vi "ActiveObjects_DynamicEvents_ProcessRepository_EndevoGoop3.vi"(0 "reference in":refnum<class>, 1 "Action(ReadRepository)":T1(ring), 5 "error in (no error)":errorcluster) -> (7 "QueueFromProcess":refnum<queue>, 9 "ProcessViRef":refnum<vi>, 11 "ProcessSyncQueue":refnum<queue>, 13 "EventFromProcess":refnum<user-event>, 14 "reference out":refnum<class>, 15 "EventsToProcess":refnum<user-event>, 17 "ProcessAlreadyStarted":bool, 19 "error out":errorcluster)   [LabVIEW 2010]
uses:
  ActiveObjects_DynamicEvents_Process.ctl
panel:
  # "Use this indicator for sending messages to the Process VI"
  # "These indicators are used by the process VIs"
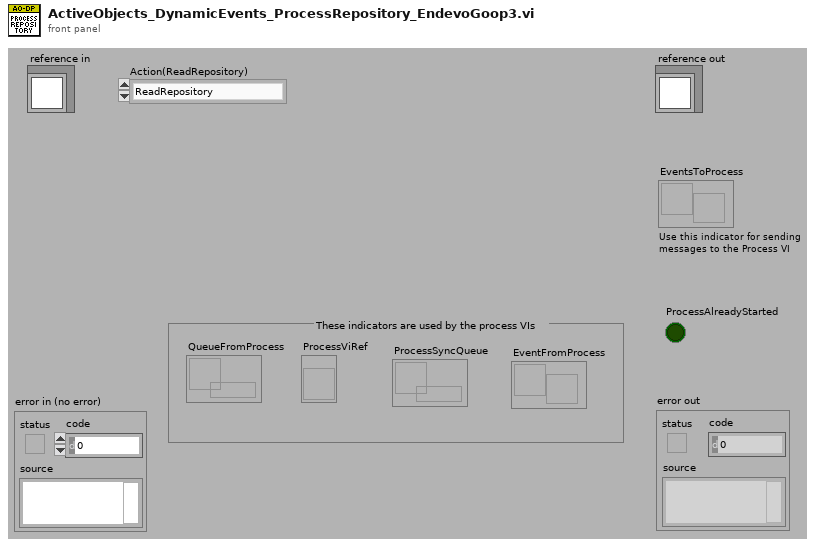
[diagram p1: front panel]
types:
  T1 = enum16{"ReadRepository", "CreateNew", "CreateOrLookUpExisting"}
  T2 = typedef "ActiveObjects_DynamicEvents_Process.ctl" = cluster{"EventsToProcess":refnum<user-event>, "EventFromProcess":refnum<user-event>, "ProcessSyncQueue":refnum<queue>, "ProcessViRef":refnum<vi>, "QueueFromProcess":refnum<queue>}
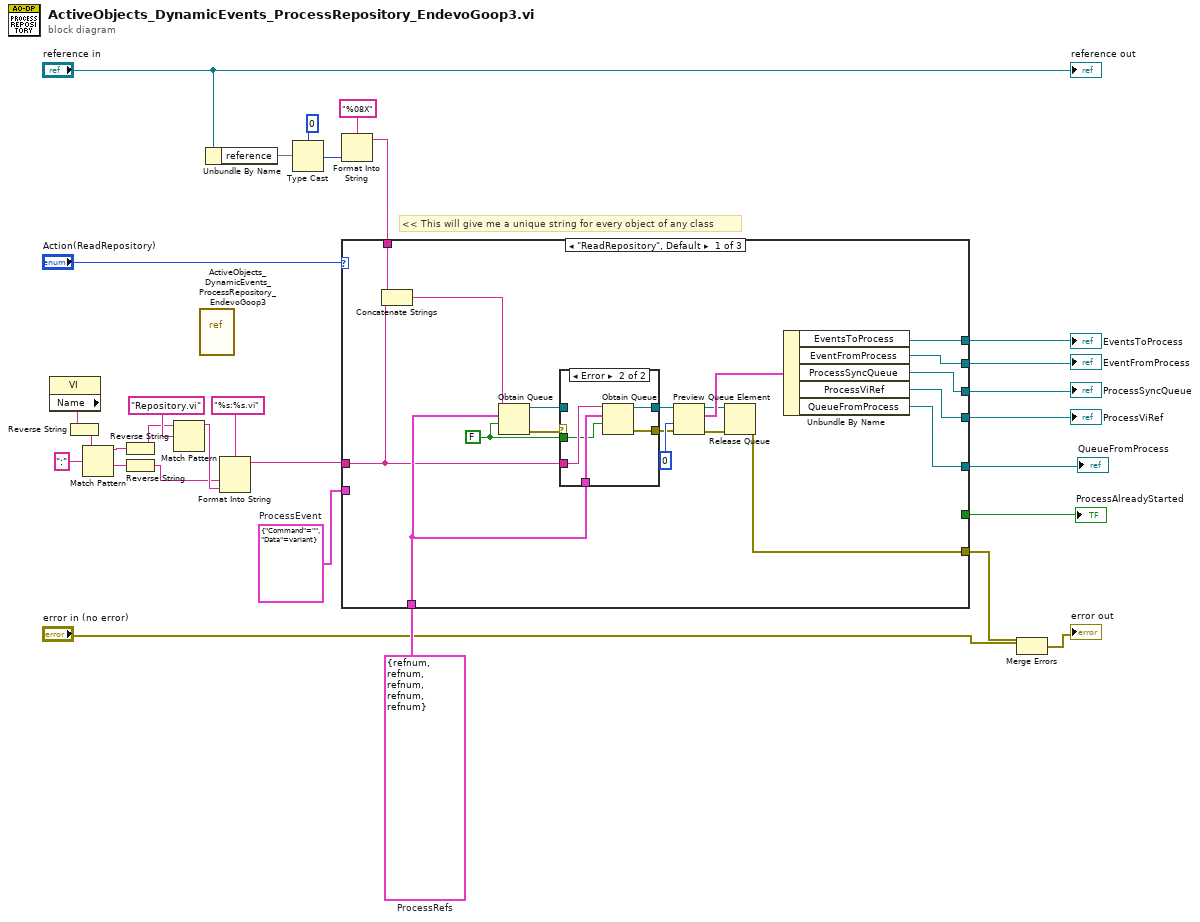
[diagram p0: block diagram]
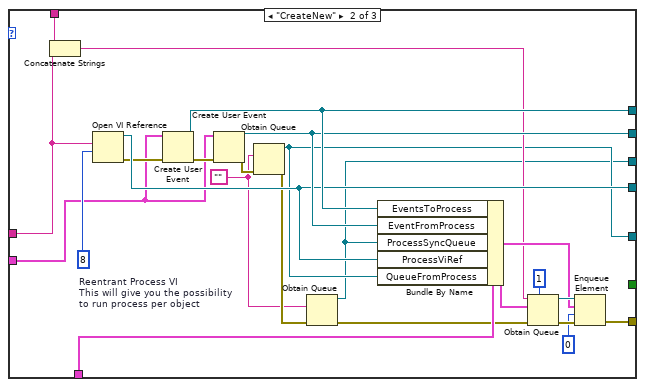
[diagram p3: hidden frame]
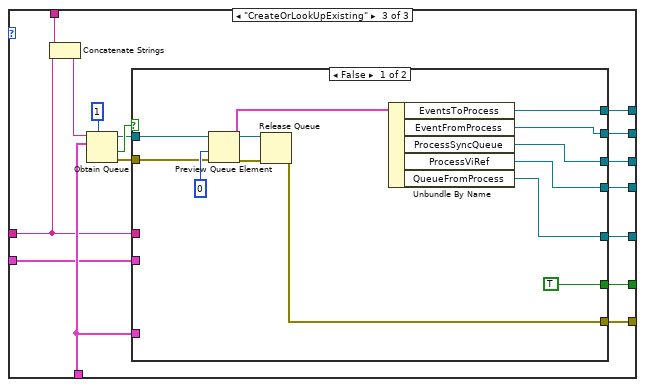
[diagram p4: hidden frame]
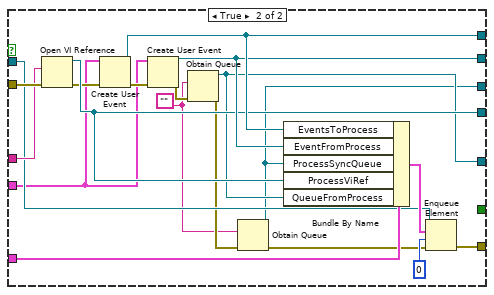
[diagram p5: hidden frame]
diagram:
  w13 = T2 {"EventsToProcess"=refnum, "EventFromProcess"=refnum, "ProcessSyncQueue"=refnum, "ProcessViRef"=refnum, "QueueFromProcess"=refnum}  # ProcessRefs
  w14 = cluster{"Command":string, "Data":variant} {"Command"="", "Data"=variant}  # ProcessEvent
  # "<< This will give me a unique string for every object of any class"
  n1 = property class="VI"() -> ("Name"=w20:string)  [unwired: 2 in, 2 out]
  n2 = Reverse String(1:w20) -> (0:w21:string)
  n3 = Match Pattern(string=w21, regular expression=":") -> (before substring=w25:string, after substring=w22:string)  [unwired: 1 in, 2 out]
  n4 = Reverse String(1:w25) -> (0:w26:string)
  n5 = Reverse String(1:w22) -> (0:w24:string)
  n6 = Match Pattern(string=w26, regular expression="Repository.vi") -> (before substring=w28:string)  [unwired: 1 in, 3 out]
  n7 = vi-ref "ActiveObjects_DynamicEvents_ProcessRepository_EndevoGoop3.vi"() -> ()  [unwired: 1 out]
  n8 = Unbundle By Name("reference in") -> ("reference"=w15)
  n9 = Format Into String(format string="%s:%s.vi", w24, w28) -> (resulting string=w3:string)  [unwired: 2 in, 1 out]
  n10 = Type Cast(type=u32 0, x=w15) -> (*(type *) &x=w18:u32)
  n11 = Format Into String(format string="%08X", w18) -> (resulting string=w5:string)  [unwired: 2 in, 1 out]
  n12 = case shown="\"ReadRepository\", Default" "Action(ReadRepository)" {
    tunnel: [w44 w56 w92] -> w8
    tunnel: [w46 w78 w94] -> w6
    tunnel: [w45 w77 w93] -> w7
    tunnel: [w47 w76 w91] -> w9
    tunnel: w13 -> [w39 w66 w87]
    tunnel: w5 -> [w37 w65 w83]
    tunnel: [w30 w75 w90] -> w11
    tunnel: w3 -> [w36 w63 w82]
    tunnel: [_ _ w85] -> w10
    tunnel: w14 -> [_ w62 w80]
    tunnel: [w34 w60 w79] -> w1
    frame "ReadRepository", Default {
      w38 = FALSE ("create if not found? (T)")
      n13 = Concatenate Strings(w37, w36) -> (w35:string)
      n14 = Obtain Queue(name (unnamed)=w35, element data type=w39, create if not found? (T)=w38) -> (queue out=w41:refnum<queue>, error out=w43:errorcluster)  [unwired: 2 in, 1 out]
      n15 = case shown="Error" w43 {
        selector: w43 -> [w50 _]
        tunnel: [w50 w52] -> w42
        tunnel: w41 -> [w49 _]
        tunnel: [w49 w53] -> w40
        tunnel: w39 -> [_ w55]
        tunnel: w36 -> [_ w54]
        tunnel: w38 -> [_ w51]
        frame No Error {
        }
        frame Error {
          n16 = Obtain Queue(name (unnamed)=w54, element data type=w55, create if not found? (T)=w51) -> (queue out=w53:refnum<queue>, error out=w52:errorcluster)  [unwired: 2 in, 1 out]
        }
      }
      n17 = Preview Queue Element(queue=w40, timeout in ms (-1)=0, error in (no error)=w42) -> (queue out=w32:refnum<queue>, element=w33:T2, error out=w31:errorcluster)  [unwired: 1 out]
      n18 = Release Queue(queue=w32, error in (no error)=w31) -> (error out=w30:errorcluster)  [unwired: 1 in, 2 out]
      n19 = Unbundle By Name(w33) -> ("EventsToProcess"=w46:refnum<user-event>, "EventFromProcess"=w45:refnum<user-event>, "ProcessSyncQueue"=w44:refnum<queue>, "ProcessViRef"=w47:refnum<vi>, "QueueFromProcess"=w34:refnum<queue>)
    }
    frame "CreateNew" {
      w57 = ""
      w72 = 8  # Reentrant Process VI This will give you the possibility to run process per object
      n20 = Concatenate Strings(w65, w63) -> (w64:string)
      n21 = Open VI Reference(vi path=w63, options=w72) -> (vi reference=w76:refnum<vi>, error out=w73:errorcluster)  [unwired: 4 in]
      n22 = Create User Event(user event datatype=w62, error in=w73) -> (user event=w78:refnum<user-event>, error out=w74:errorcluster)
      n23 = Create User Event(user event datatype=w62, error in=w74) -> (user event=w77:refnum<user-event>, error out=w61:errorcluster)
      n24 = Obtain Queue(element data type=w57, error in (no error)=w61) -> (queue out=w60:refnum<queue>, error out=w59:errorcluster)  [unwired: 3 in, 1 out]
      n25 = Obtain Queue(element data type=w57, error in (no error)=w59) -> (queue out=w56:refnum<queue>, error out=w58:errorcluster)  [unwired: 3 in, 1 out]
      n26 = Bundle By Name(cluster=w66, "EventsToProcess"=w78, "EventFromProcess"=w77, "ProcessSyncQueue"=w56, "ProcessViRef"=w76, "QueueFromProcess"=w60) -> (w69:T2)
      n27 = Obtain Queue(max queue size (-1, unlimited)=1, name (unnamed)=w64, element data type=w69, error in (no error)=w58) -> (queue out=w71:refnum<queue>, error out=w70:errorcluster)  [unwired: 1 in, 1 out]
      n28 = Enqueue Element(queue=w71, element=w69, timeout in ms (-1)=0, error in (no error)=w70) -> (error out=w75:errorcluster)  [unwired: 2 out]
    }
    frame "CreateOrLookUpExisting" {
      n29 = Concatenate Strings(w83, w82) -> (w81:string)
      n30 = Obtain Queue(max queue size (-1, unlimited)=1, name (unnamed)=w81, element data type=w87) -> (queue out=w88:refnum<queue>, created new?=w89:bool, error out=w86:errorcluster)  [unwired: 2 in]
      n31 = case shown="False" w89 {
        tunnel: [w107 w126] -> w94
        tunnel: [w106 w125] -> w93
        tunnel: [w105 w108] -> w92
        tunnel: [w104 w124] -> w91
        tunnel: [w95 w123] -> w90
        tunnel: w87 -> [_ w122]
        tunnel: w86 -> [w101 w117]
        tunnel: w82 -> [_ w116]
        tunnel: w88 -> [w102 w115]
        tunnel: [TRUE _] -> w85
        tunnel: w80 -> [_ w114]
        tunnel: [w98 w112] -> w79
        frame False {
          n32 = Preview Queue Element(queue=w102, timeout in ms (-1)=0, error in (no error)=w101) -> (queue out=w97:refnum<queue>, element=w100:T2, error out=w96:errorcluster)  [unwired: 1 out]
          n33 = Release Queue(queue=w97, error in (no error)=w96) -> (error out=w95:errorcluster)  [unwired: 1 in, 2 out]
          n34 = Unbundle By Name(w100) -> ("EventsToProcess"=w107:refnum<user-event>, "EventFromProcess"=w106:refnum<user-event>, "ProcessSyncQueue"=w105:refnum<queue>, "ProcessViRef"=w104:refnum<vi>, "QueueFromProcess"=w98:refnum<queue>)
        }
        frame True {
          w109 = ""
          n35 = Open VI Reference(vi path=w116, error in (no error)=w117) -> (vi reference=w124:refnum<vi>, error out=w120:errorcluster)  [unwired: 4 in]
          n36 = Create User Event(user event datatype=w114, error in=w120) -> (user event=w126:refnum<user-event>, error out=w121:errorcluster)
          n37 = Create User Event(user event datatype=w114, error in=w121) -> (user event=w125:refnum<user-event>, error out=w113:errorcluster)
          n38 = Obtain Queue(element data type=w109, error in (no error)=w113) -> (queue out=w112:refnum<queue>, error out=w111:errorcluster)  [unwired: 3 in, 1 out]
          n39 = Obtain Queue(element data type=w109, error in (no error)=w111) -> (queue out=w108:refnum<queue>, error out=w110:errorcluster)  [unwired: 3 in, 1 out]
          n40 = Bundle By Name(cluster=w122, "EventsToProcess"=w126, "EventFromProcess"=w125, "ProcessSyncQueue"=w108, "ProcessViRef"=w124, "QueueFromProcess"=w112) -> (w119:T2)
          n41 = Enqueue Element(queue=w115, element=w119, timeout in ms (-1)=0, error in (no error)=w110) -> (error out=w123:errorcluster)  [unwired: 2 out]
        }
      }
    }
  }
  "ProcessSyncQueue" <- w8
  "EventsToProcess" <- w6
  "EventFromProcess" <- w7
  "ProcessViRef" <- w9
  "ProcessAlreadyStarted" <- w10
  "QueueFromProcess" <- w1
  n42 = Merge Errors("error in (no error)", w11) -> (→"error out":errorcluster)
  "reference out" <- "reference in"
